vi "Python-1.vi"() -> ()   [LabVIEW 2020]
doc: "This example demonstrates how to call a Python function and pass doubles as arguments. It uses a python function to compute the sum of two doubles."
panel:
  in  "stop":bool
  out "module path":path
  out "error out":errorcluster
  out "a + b":dbl
  in  "b":dbl=1.0
  in  "a":dbl=41.0
  in  "error in (no error)":errorcluster
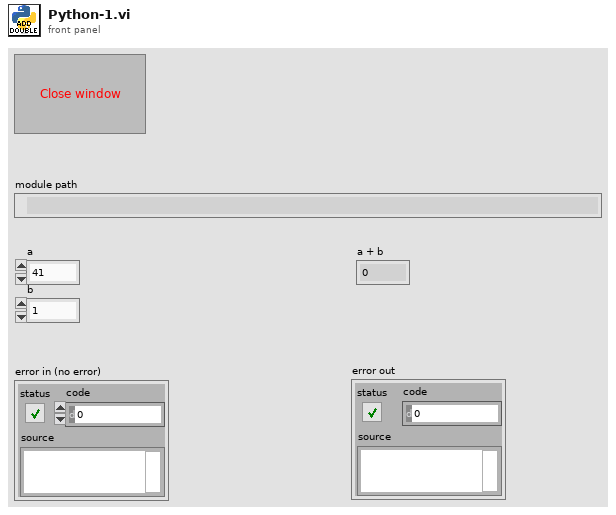
[diagram p1: front panel]
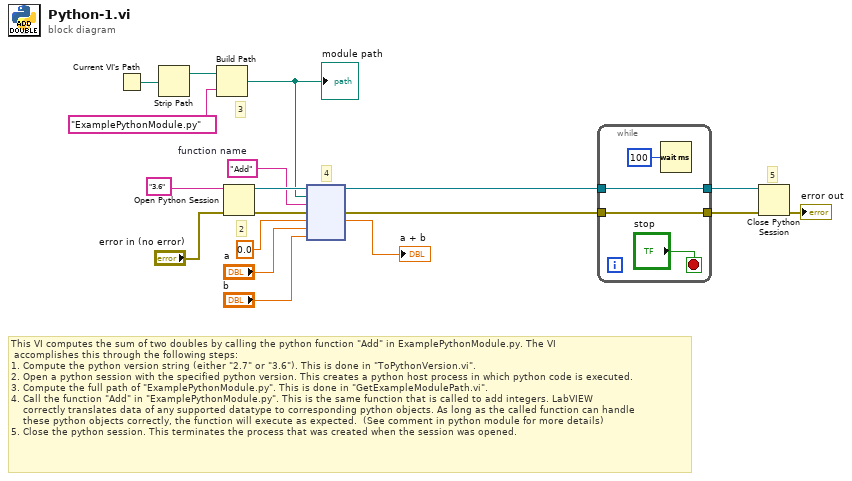
[diagram p0: block diagram]
diagram:
  w15 = "Add"  # function name
  # "5"
  # "4"
  # "2"
  # "3"
  # "This VI computes the sum of two doubles by calling the python function \"Add\" in ExamplePythonModule.py. The VI\n accomplishes this through the following steps:\n1. Compute the python version string (either \"2.7\" or \"3.6\"). This is done in \"ToPythonVersion.vi\". \n2. Open a python session with the specified python version. This creates a python host process in which python code is executed.\n3. Compute the full path of \"ExamplePythonModule.py\". This is done in \"GetExampleModulePath.vi\".\n4. Call the function \"Add\" in \"ExamplePythonModule.py\". This is the same function that is called to add integers. LabVIEW \n    correctly translates data of any supported datatype to corresponding python objects. As long as the called function can handle\n    these python objects correctly, the function will execute as expected.  (See comment in python module for more details)\n5. Close the python session. This terminates the process that was created when the session was opened."
  n1 = Current VI's Path() -> (path=w9:path)
  n2 = Strip Path(path=w9) -> (stripped path=w8:path)  [unwired: 1 out]
  n3 = Build Path(base path=w8, name or relative path="ExamplePythonModule.py") -> (appended path=w6:path)
  "module path" <- w6
  n4 = Open Python Session(python version="3.6" ("Python version"), 3:"error in (no error)") -> (session out=w17:refnum<k35>, error out=w16:errorcluster)  [unwired: 1 in]
  n5 = node(w17, w6, w15, w16, 0.0 ("a"), "a", "b") -> (w4:refnum<k35>, w2:errorcluster, →"a + b":dbl)  [unwired: 2 in, 2 out]
  n6 = while {
    tunnel: [w21] -> w5
    tunnel: w4 -> [w21]
    tunnel: [w20] -> w3
    tunnel: w2 -> [w20]
    stop <- "stop" stop-if-true
    n7 = Wait (ms)(milliseconds to wait=u32 100) -> ()  [unwired: 1 out]
  }
  n8 = Close Python Session(session in=w5, error in=w3) -> (11:→"error out":errorcluster)
